vi "Basic trigo.vi"(2 "Distance from camera":dbl, 3 "Camera offset Y":dbl, 4 "Caamera offset X":dbl) -> (0 "Delta hieght":dbl, 1 "Distance on ground":dbl)   [LabVIEW 2012]
uses:
  Motors Values.vi
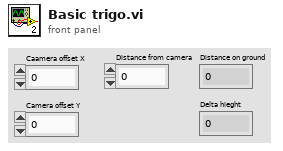
[diagram p1: front panel]
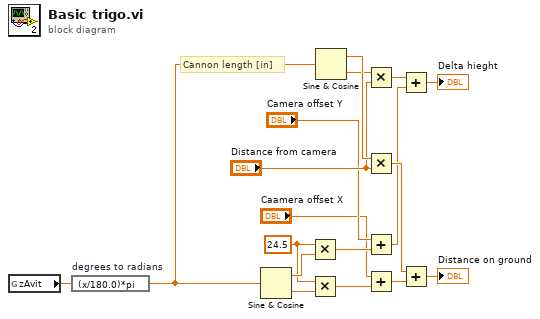
[diagram p0: block diagram]
diagram:
  w17 = 24.5
  # "Cannon length [in]"
  n1 = global read "Motors Values.vi" "zAvit"() -> (w15:dbl)
  n2 = expression code="(x/180.0)*pi" "degrees to radians"(w15) -> (w14:dbl)
  n3 = Sine & Cosine(0:w14) -> (1:w18:dbl, 2:w16:dbl)
  n4 = Multiply(x=w17, y=w18) -> (x*y=w9:dbl)
  n5 = Multiply(x=w17, y=w16) -> (x*y=w4:dbl)
  n6 = Sine & Cosine(0:w14) -> (1:w13:dbl, 2:w12:dbl)
  n7 = Multiply(x=w12, y="Distance from camera") -> (x*y=w5:dbl)
  n8 = Multiply(x=w13, y="Distance from camera") -> (x*y=w6:dbl)
  n9 = Add(x="Camera offset Y", y=w9) -> (x+y=w1:dbl)
  n10 = Add(x="Caamera offset X", y=w4) -> (x+y=w2:dbl)
  n11 = Add(x=w5, y=w1) -> (x+y=→"Delta hieght":dbl)
  n12 = Add(x=w6, y=w2) -> (x+y=→"Distance on ground":dbl)
